vi "dll.midi_file_close.vi"(8 "error in (no error)":errorcluster, 11 "midi file in":refnum<class "midi file.lvclass">) -> (0 "error out":errorcluster, 3 "midi file out":refnum<class "midi file.lvclass">)   [LabVIEW 2020, in "MIDIllan.lvlib" / "midi file.lvclass"]
uses:
  midi file.lvclass
  midi file.lvclass/midi file.ctl
  MIDIllan/MIDIllan.lvlib
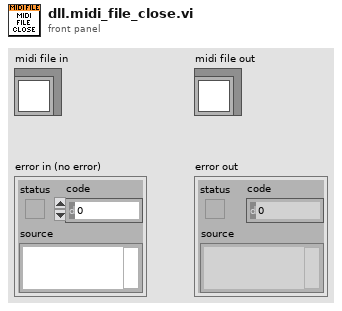
[diagram p1: front panel]
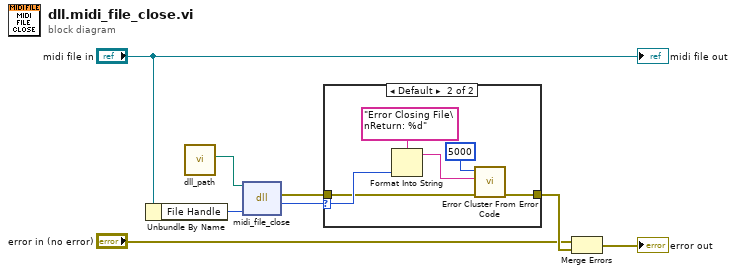
[diagram p0: block diagram]
diagram:
  n1 = Unbundle By Name("midi file in") -> ("File Handle"=w1:i32)
  n2 = call "dll_path.vi"() -> ("dll"=w8:path)  [unwired: 11 in]
  n3 = dll-call lib="C:/code/LabVIEW-MIDI-XPLAT/dist/TomMIDIllan_*.*" fn="midi_file_close"(path in=w8, "File Handle"=w1) -> (error out=w7:errorcluster, "Error code"=w6:i32)  [unwired: 3 in, 1 out]
  n4 = case shown="Default" w6 {
    selector: w6 -> [_ w12]
    tunnel: w7 -> [w9 w11]
    tunnel: [w9 w10] -> w4
    frame 0.. {
    }
    frame Default {
      n5 = Format Into String(format string="Error Closing File\nReturn: %d", w12) -> (resulting string=w13:string)  [unwired: 2 in, 1 out]
      n6 = call <vilib>:"Error Cluster From Error Code.vi"("error in (no error)"=w11, "error message (\"\")"=w13, "error code (0)"=5000) -> ("error out"=w10:errorcluster)  [unwired: 6 in]
    }
  }
  n7 = Merge Errors("error in (no error)", w4) -> (→"error out":errorcluster)
  "midi file out" <- "midi file in"
